vi "Scroll-Vzoom.vi"(8 "error in (no error)":errorcluster, 9 "Scroll value":i32, 10 "Coords":T1, 11 "Gviewer in":refnum<class "Gviewer.lvclass">) -> (0 "error out":errorcluster, 3 "Gviewer out":refnum<class "Gviewer.lvclass">)   [LabVIEW 2020, in "Gviewer.lvclass"]
doc: "Andre Koelewijn, 31 jan 2021\n\nVertically zoom Y-axis using the mouse scroll wheel"
uses:
  Gviewer.lvclass
  <vilib>/Utility/miscctls.llb/LVPoint32TypeDef.ctl
  Gviewer.lvclass/Gviewer.ctl
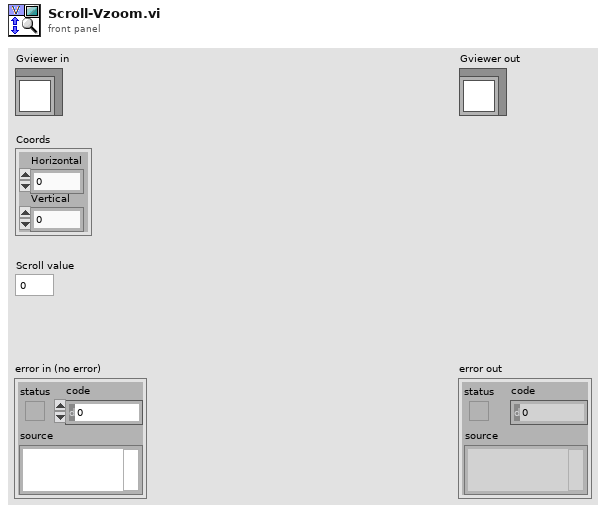
[diagram p1: front panel]
types:
  T1 = typedef "LVPoint32TypeDef.ctl" = cluster{"Horizontal":i32, "Vertical":i32}
  T2 = typedef "Gviewer.lvclass/Typedef_SelProperties.ctl" = cluster{"Color":u32, "LineType":T3, "max":dbl, "min":dbl}
  T3 = typedef "Gviewer.lvclass/Typedef_LineType.ctl" = enum16{"num_bare", "num_MinMax_Area", "num_MinMax_Lines", "num_MinMax_Forfor", "num_Max_Area", "num_Max_Line", "num_Max_Forfor", "num_Min_Area", "num_Min_Line", "num_Min_Fosfor", "Boolean_Line_01", "Boolean_Area_01", "Boolean_Fosfor_01", "Boolean_Line_TF", "Boolean_Area_TF", "Boolean_Fosfor_TF", "Boolean_OnOff_Line", "Boolean_OnOff_Area", "Boolean_OnOff_Fosfor", "Boolean_spare", "StringEvent_Line", "StringEvent_TimeLine"}
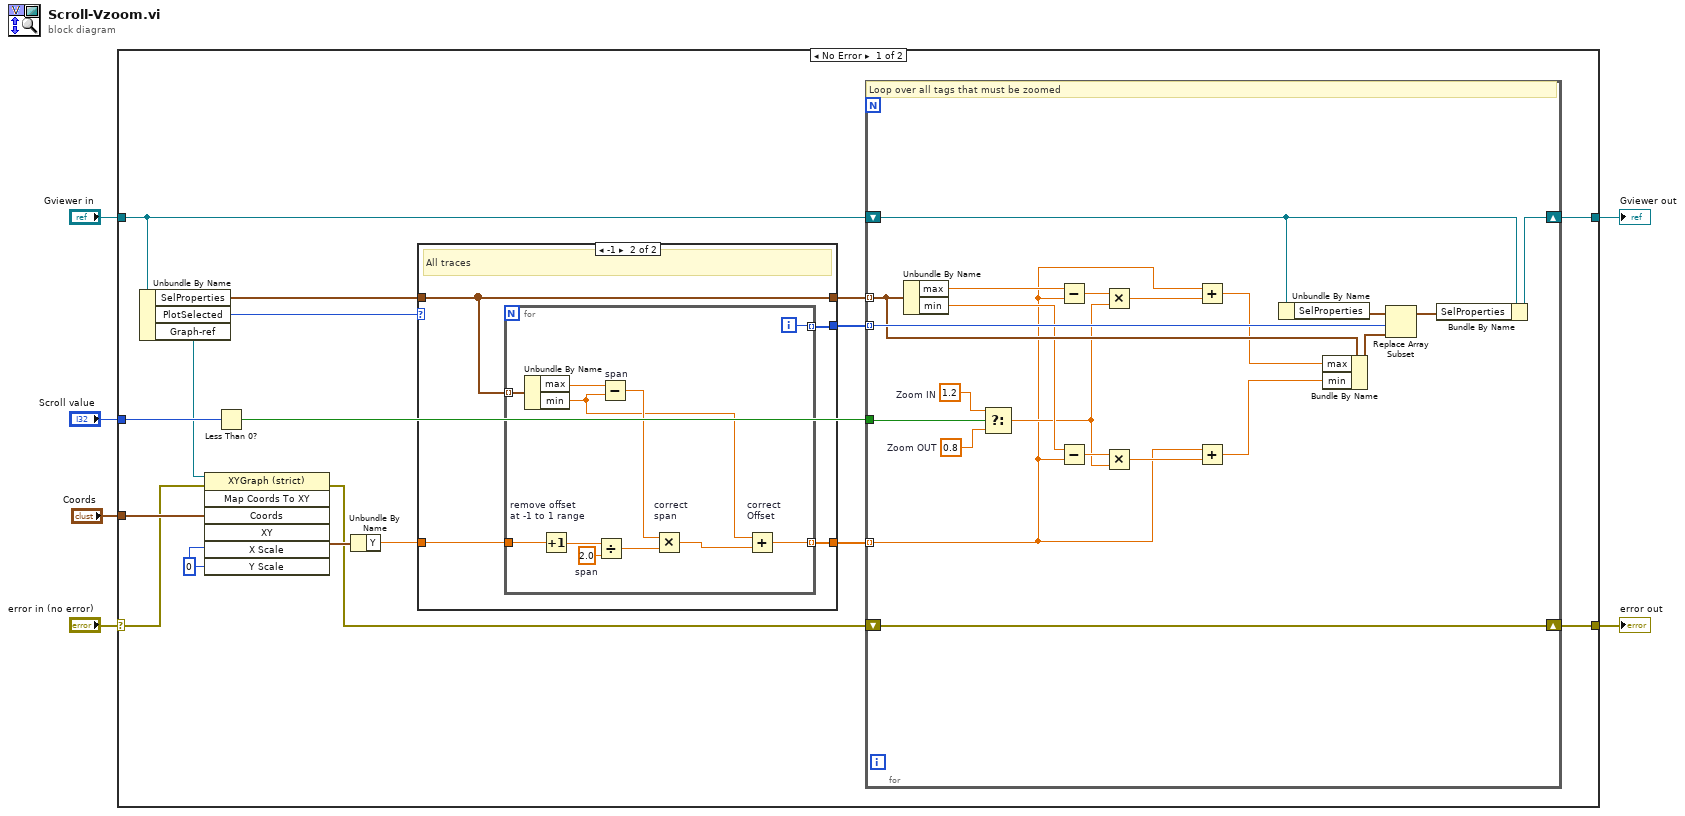
[diagram p0: block diagram]
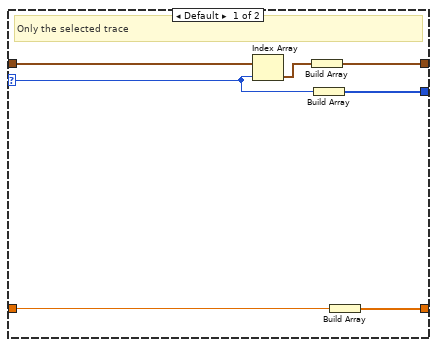
[diagram p2: hidden frame]
diagram:
  n1 = case shown="No Error" "error in (no error)" {
    selector: "error in (no error)" -> [w11 w68]
    tunnel: [w19 w68] -> w5
    tunnel: [w20 w67] -> w3
    tunnel: "Gviewer in" -> [w21 w67]
    tunnel: "Scroll value" -> [w17 _]
    tunnel: "Coords" -> [w13 _]
    frame No Error {
      w15 = 0 ("Y Scale")
      n2 = Unbundle By Name(w21) -> ("SelProperties"=w22:T2[], "PlotSelected"=w23:i32, "Graph-ref"=w12:refnum<vi>)
      n3 = invoke class="XYGraph (strict)" method="Map Coords To XY"(reference=w12, error in=w11, "Coords"=w13, "X Scale"=w15, "Y Scale"=w15) -> (error out=w10:errorcluster, "XY"=w14:cluster{"X":dbl, "Y":dbl})  [unwired: 2 in, 5 out]
      n4 = Less Than 0?(x=w17) -> (x < 0?=w16:bool)
      n5 = Unbundle By Name(w14) -> ("Y"=w8:dbl)
      n6 = case shown="-1" w23 {
        selector: w23 -> [w48 _]
        tunnel: w22 -> [w50 w54]
        tunnel: [w51 w54] -> w18
        tunnel: [w47 w55] -> w9
        tunnel: w8 -> [w46 w53]
        tunnel: [w45 w52] -> w7
        frame Default {
          # "Only the selected trace"
          n7 = Index Array(array=w50, index=w48) -> (element=w49:T2)
          n8 = Build Array(w49) -> (w51:T2[])
          n9 = Build Array(w48) -> (w47:i32[])
          n10 = Build Array(w46) -> (w45:dbl[])
        }
        frame -1 {
          # "All traces"
          n11 = for {
            tunnel: [w66] -> w55 mode=indexing
            tunnel: w54 -> [w65] mode=indexing
            tunnel: w53 -> [w63]
            tunnel: [w56] -> w52 mode=indexing
            i -> [w66]
            w61 = 2.0  # span
            n12 = Unbundle By Name(w65) -> ("max"=w64:dbl, "min"=w57:dbl)
            n13 = Increment "remove offset\nat -1 to 1 range"(x=w63) -> (x+1=w62:dbl)
            n14 = Divide(x=w62, y=w61) -> (x/y=w60:dbl)
            n15 = Subtract "span"(x=w64, y=w57) -> (x-y=w59:dbl)
            n16 = Multiply "correct\nspan"(x=w59, y=w60) -> (x*y=w58:dbl)
            n17 = Add "correct\nOffset"(x=w57, y=w58) -> (x+y=w56:dbl)
          }
        }
      }
      n18 = for {
        shift-right: [w37] -> w20
        shift-left: w21 -> [w38]
        shift-right: [w44] -> w19
        shift-left: w10 -> [w44]
        tunnel: w18 -> [w35] mode=indexing
        tunnel: w16 -> [w43]
        tunnel: w7 -> [w24] mode=indexing
        tunnel: w9 -> [w36] mode=indexing
        w41 = 0.8  # Zoom OUT
        w42 = 1.2  # Zoom IN
        # "Loop over all tags that must be zoomed"
        n19 = Unbundle By Name(w35) -> ("max"=w32:dbl, "min"=w28:dbl)
        n20 = Select(t=w42, s=w43, f=w41) -> (s? t:f=w27:dbl)
        n21 = Subtract(x=w32, y=w24) -> (x-y=w33:dbl)
        n22 = Subtract(x=w28, y=w24) -> (x-y=w29:dbl)
        n23 = Multiply(x=w33, y=w27) -> (x*y=w25:dbl)
        n24 = Multiply(x=w29, y=w27) -> (x*y=w30:dbl)
        n25 = Add(x=w24, y=w25) -> (x+y=w31:dbl)
        n26 = Add(x=w24, y=w30) -> (x+y=w26:dbl)
        n27 = Unbundle By Name(w38) -> ("SelProperties"=w40:T2[])
        n28 = Bundle By Name(cluster=w35, "max"=w31, "min"=w26) -> (w34:T2)
        n29 = Replace Array Subset(array=w40, new element=w34, index=w36) -> (w39:T2[])
        n30 = Bundle By Name(cluster=w38, "SelProperties"=w39) -> (w37:refnum<class "Gviewer.lvclass">)
      }
    }
    frame Error {
    }
  }
  "error out" <- w5
  "Gviewer out" <- w3
